vi "ParseMsgAnalogIO.vi"(8 "error in":errorcluster, 11 "Sysex Message":u8[](array[numeric]) format="%x") -> (0 "error out":errorcluster, 3 "AnalogADCValues":u16[](array[numeric]))   [LabVIEW 2020, in "FirmataClient.lvlib"]
doc: "Parse a message according to the Firmata Protocol Requirements. \n- https://github.com/firmata/protocol\n- https://github.com/firmata/protocol/blob/master/protocol.md"
uses:
  FirmataClient.lvlib
  controls/FirmataProtocolConstants.ctl
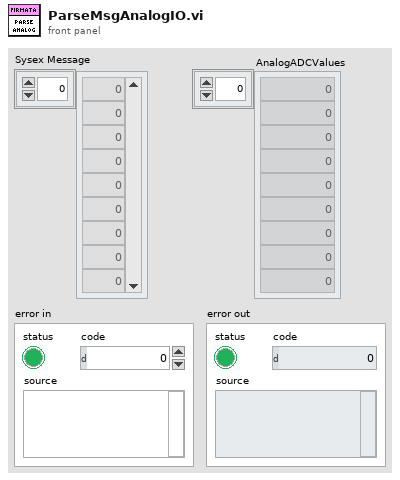
[diagram p1: front panel]
types:
  T1 = typedef "FirmataClient.lvlib/FirmataProtocolConstants.ctl" = u16
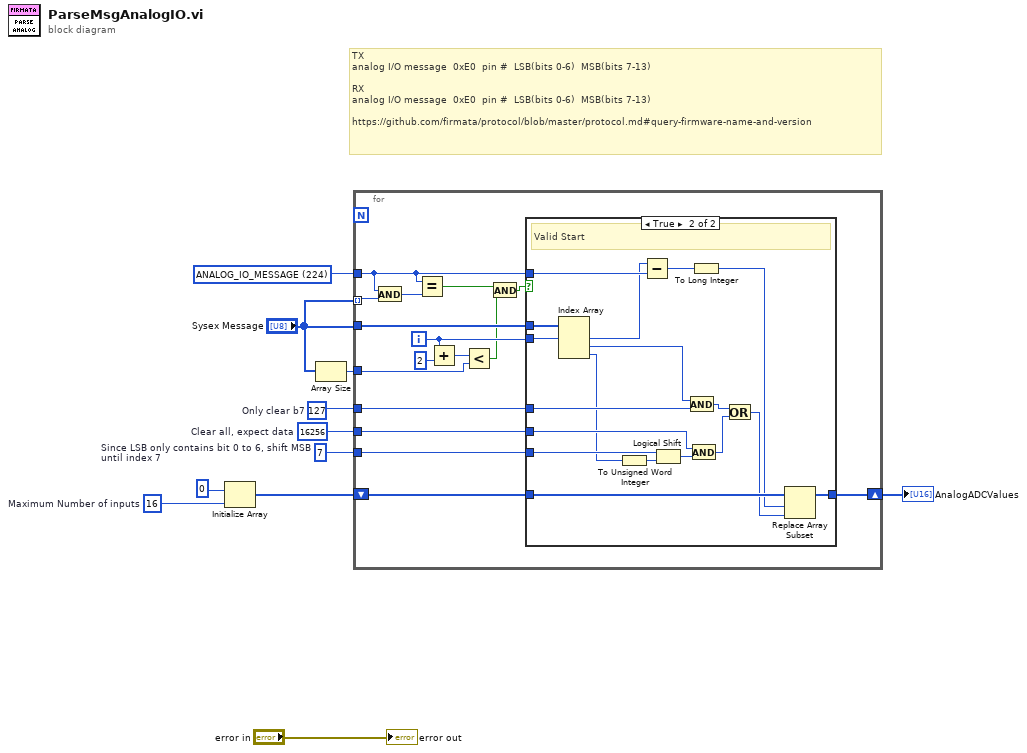
[diagram p0: block diagram]
diagram:
  w1 = T1 224 items=["ANALOG_IO_MESSAGE"=224, "DIGITAL_IO_MESSAGE"=144, "REPORT_ANALOG_PIN"=192, "REPORT_DIGITAL_PORT"=208, "START_SYSEX"=240, "END_SYSEX"=247, "SET_PIN_MODE"=244, "SET_DIGITAL_PIN_VALUE"=245, "PROTOCOL_VERSION"=249, "SYSTEM_RESET"=255, "SYSEX.EXTENDED_ID"=0, "SYSEX.RESERVED_USER_COMMANDs"=1, "SYSEX.ANALOG_MAPPING_QUERY"=105, "SYSEX.ANALOG_MAPPING_RESPONSE"=106, "SYSEX.CAPABILITY_QUERY"=107, "SYSEX.CAPABILITY_RESPONSE"=108, "SYSEX.PIN_STATE_QUERY"=109, "SYSEX.PIN_STATE_RESPONSE"=110, "SYSEX.REPORT_FIRMWARE"=121, "SYSEX.EXTENDED_ANALOG"=111, "SYSEX.STRING_DATA"=113, "SYSEX.REALTIME"=127, "SYSEX.NON_REALTIME"=126, "SYSEX.SAMPLING_INTERVAL"=122] ("FimataProtocolConstants")
  w6 = i16 16  # Maximum Number of inputs
  w8 = u8 127  # Only clear b7
  w9 = u16 16256  # Clear all, expect data
  w10 = i16 7  # Since LSB only contains bit 0 to 6, shift MSB until index 7
  # "TX\nanalog I/O message \t0xE0 \tpin # \tLSB(bits 0-6) \tMSB(bits 7-13)\n\nRX\nanalog I/O message \t0xE0 \tpin # \tLSB(bits 0-6) \tMSB(bits 7-13)\n\nhttps://github.com/firmata/protocol/blob/master/protocol.md#query-firmware-name-and-version"
  n1 = Initialize Array(u16 0 ("dimension size"), w6) -> (w5:u16[])
  n2 = Array Size(array="Sysex Message") -> (size(s)=w2:i32)
  n3 = for {
    tunnel: w1 -> [w21]
    tunnel: "Sysex Message" -> [w27] mode=indexing
    tunnel: "Sysex Message" -> [w25]
    tunnel: w10 -> [w24]
    tunnel: w9 -> [w23]
    tunnel: w8 -> [w22]
    shift-right: [w19] -> w4
    shift-left: w5 -> [w20]
    tunnel: w2 -> [w15]
    i -> [w18]
    n4 = And(x=w21, y=w27) -> (x .and. y?=w26:T1)
    n5 = Equal?(x=w21, y=w26) -> (x = y?=w14:bool)
    n6 = Add(x=w18, y=2) -> (x+y=w16:i32)
    n7 = Less?(x=w16, y=w15) -> (x < y?=w13:bool)
    n8 = And(x=w14, y=w13) -> (x .and. y?=w12:bool)
    n9 = case shown="True" w12 {
      tunnel: w25 -> [_ w46]
      tunnel: w18 -> [_ w45]
      tunnel: w24 -> [_ w43]
      tunnel: w23 -> [_ w41]
      tunnel: w22 -> [_ w39]
      tunnel: w21 -> [_ w35]
      tunnel: w20 -> [w28 w33]
      tunnel: [w28 w32] -> w19
      frame False {
      }
      frame True {
        # "Valid Start"
        n10 = Index Array(array=w46, index #1=w45) -> (element #1=w34:u8, element #2=w36:u8, element #3=w37:u8)  [unwired: 2 in]
        n11 = To Unsigned Word Integer(number=w37) -> (unsigned 16bit integer=w44:u16)
        n12 = Subtract(x=w34, y=w35) -> (x-y=w30:T1)
        n13 = Logical Shift(y=w43, x=w44) -> (x << y=w42:u16)
        n14 = And(x=w36, y=w39) -> (x .and. y?=w38:u8)
        n15 = And(x=w41, y=w42) -> (x .and. y?=w40:u16)
        n16 = To Long Integer(number=w30) -> (32bit integer=w29:i32)
        n17 = Or(x=w38, y=w40) -> (x .or. y?=w31:u16)
        n18 = Replace Array Subset(array=w33, new element=w31, index=w29) -> (w32:u16[])
      }
    }
  }
  "AnalogADCValues" <- w4
  "error out" <- "error in"
